vi "Set NRD wrapper.vi"(0 "dwDevIndex":u32, 1 "bAckEna":i32, 2 "dOut":string, 5 "dwCanNodeId":u32, 7 "uiDCIn":u32, 9 "dIn":string, 11 "error in (no error)":errorcluster caption="错误输入（无错误）", 12 "uiDCOut":u32) -> (4 "dOut out":string, 6 "function return":u32, 10 "dIn out":string, 15 "error out":errorcluster caption="错误输出")   [LabVIEW 2016, in "UISimCanFunc_wrapper.lvlib"]
doc: "_declspec (dllexport) DWORD SetNRD_wrapper(DWORD dwDevIndex, DWORD dwCanNodeId, UINT uiDCIn, UCHAR dIn[6],\n BOOL bAckEna, UINT uiDCOut, UCHAR dOut[6]);"
uses:
  <userlib>/UISimCanFunc_wrapper/UISimCanFunc_wrapper.lvlib
  <userlib>/UISimCanFunc_wrapper/UISimCanFunc_wrapper.dll
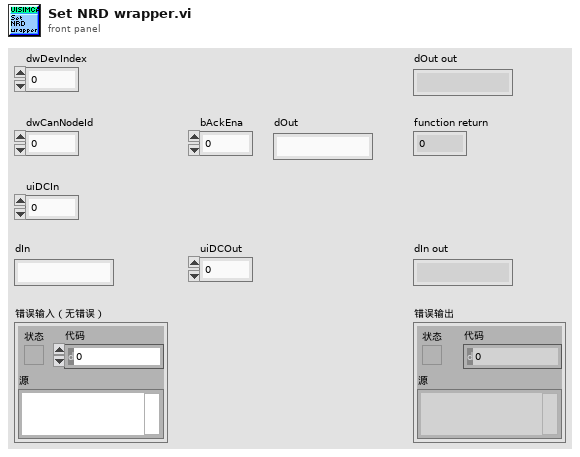
[diagram p1: front panel]
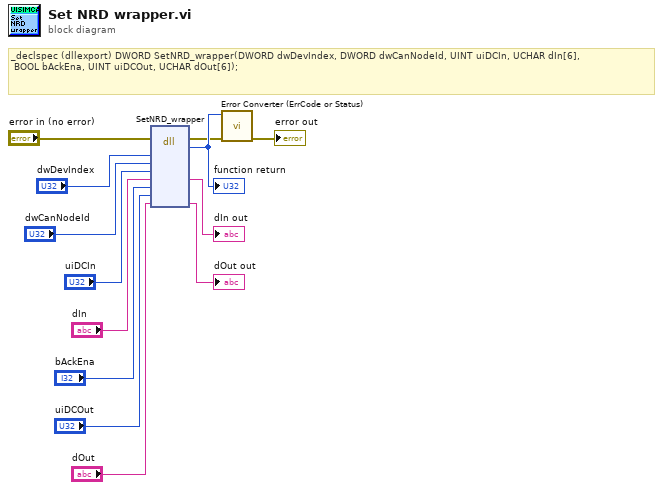
[diagram p0: block diagram]
diagram:
  # "_declspec (dllexport) DWORD SetNRD_wrapper(DWORD dwDevIndex, DWORD dwCanNodeId, UINT uiDCIn, UCHAR dIn[6],\n\tBOOL bAckEna, UINT uiDCOut, UCHAR dOut[6]);"
  n1 = dll-call lib="C:/Program Files (x86)/National Instruments/LabVIEW 2016/user.lib/UISimCanFunc_wrapper/UISimCanFunc_wrapper.*" fn="SetNRD_wrapper"(error in="error in (no error)", "dwDevIndex"="dwDevIndex", "dwCanNodeId"="dwCanNodeId", "uiDCIn"="uiDCIn", "dIn"="dIn", "bAckEna"="bAckEna", "uiDCOut"="uiDCOut", "dOut"="dOut") -> (error out=w2:errorcluster, w13:u32, "dIn"=→"dIn out":string, "dOut"=→"dOut out":string)  [unwired: 7 in, 1 out]
  "function return" <- w13
  n2 = call <userlib>:"Error Converter (ErrCode or Status).vi"("error in (no error)"=w2, "error code"=w13) -> ("error out"=→"error out":errorcluster)  [unwired: 9 in]
